vi "Pick Text Color.vi"(11 "color":u32(colorbox)) -> (2 "light?":bool, 3 "text":u32(colorbox))   [LabVIEW 2021, in "Theme.lvclass"]
doc: "perform a calculation to determine which font color should be used for a given background color\n\n<b>Code Developed By:</b> +\nDaniel Coons +\nhttps://github.com/danielcoons/tsc-pop-up"
uses:
  Theme.lvclass
  Theme.lvclass/Theme.ctl
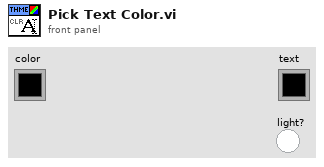
[diagram p1: front panel]
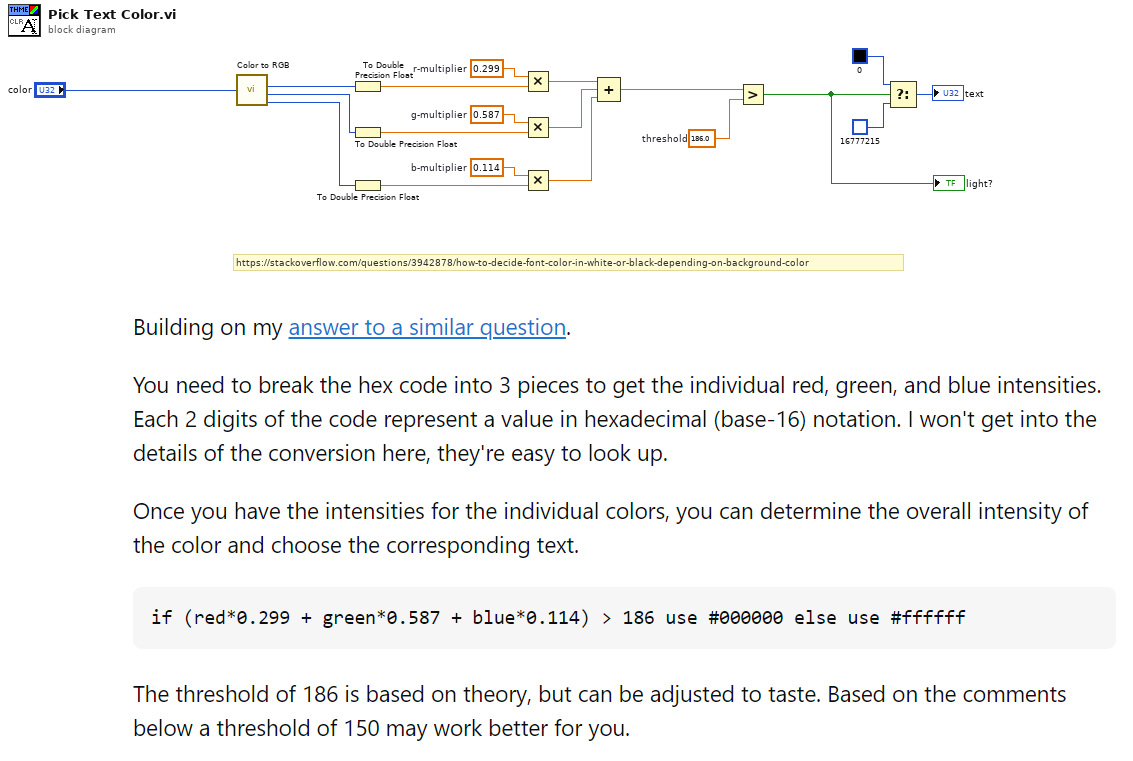
[diagram p0: block diagram]
diagram:
  w1 = 186.0  # threshold
  w6 = 0.114  # b-multiplier
  w7 = 0.587  # g-multiplier
  w8 = 0.299  # r-multiplier
  # "https://stackoverflow.com/questions/3942878/how-to-decide-font-color-in-white-or-black-depending-on-background-color"
  n1 = call <vilib>:"Color to RGB.vi"("Color"="color") -> ("R"=w18:u8, "G"=w10:u8, "B"=w9:u8)  [unwired: 1 out]
  n2 = To Double Precision Float(number=w18) -> (double precision float=w17:dbl)
  n3 = To Double Precision Float(number=w10) -> (double precision float=w16:dbl)
  n4 = To Double Precision Float(number=w9) -> (double precision float=w15:dbl)
  n5 = Multiply(x=w8, y=w17) -> (x*y=w5:dbl)
  n6 = Multiply(x=w7, y=w16) -> (x*y=w4:dbl)
  n7 = Multiply(x=w6, y=w15) -> (x*y=w3:dbl)
  n8 = Compound Arithmetic op=ADD(w5, w4, w3) -> (w2:dbl)
  n9 = Greater?(x=w2, y=w1) -> (0:w14:bool)
  "light?" <- w14
  n10 = Select(t=u32 0, s=w14, f=u32 16777215) -> (s? t:f=→"text":u32)
